vi "qDRC.vi"(0 "System no.":i32=1 min=1 max=4 step=1, 2 "Rec. table to query":i32[](array[numeric]), 3 "With Rec. table IDs?":bool, 5 "error in":errorcluster) -> (14 "Rec. option":i32[](array[numeric]), 15 "Source ID":string[](array[string]), 16 "Trigger option":i32[](array[numeric]), 19 "error out":errorcluster)   [LabVIEW 2020]
doc: "Returns the data recording configuration (Source ID and Rec. option) for the queried record table. \nGCS 2.0: Trigger option is not valid.\n\nC-413, C-843, C-866. C-867, C-877, C-886, C-887, C-891, E-517,E-518,E-709, E-712, E-725, E-727, E-753, E-754, E-861, E-871, E-873, E-874, F-206, M-8X0, Mercury_GCS: Trigger option is not valid.\n\nC-887, F-206, M-8X0: Only for GCS syntax version = GCS 2.0 or higher (check with CSV?.vi. If CSV?.vi is not supported, syntax version is GCS 1.0)."
panel:
  # "Returns the data recording configuration (Source ID, Rec. option and Trigger opt.) for the queried \nrecord tables. GCS 2.0: Trigger option is not valid."
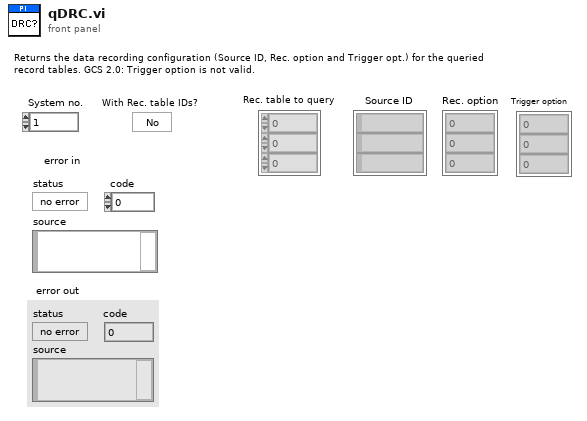
[diagram p1: front panel]
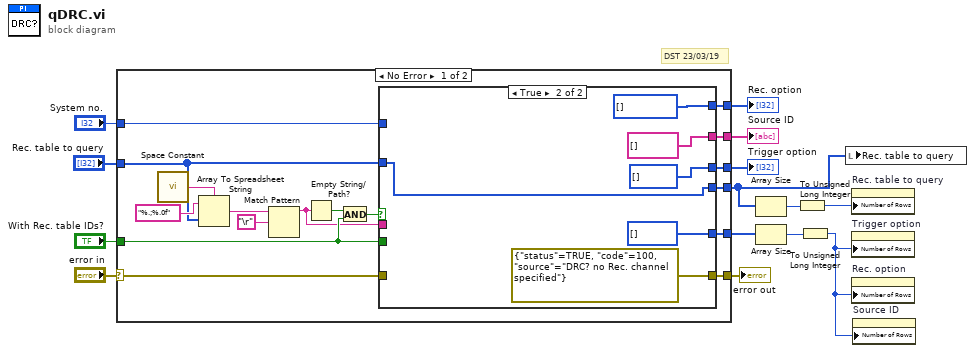
[diagram p0: block diagram]
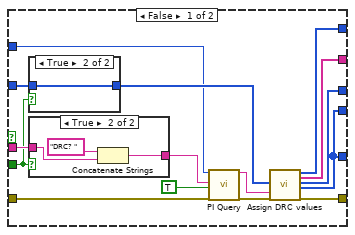
[diagram p2: hidden frame]
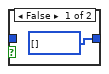
[diagram p3: hidden frame]
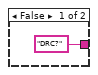
[diagram p4: hidden frame]
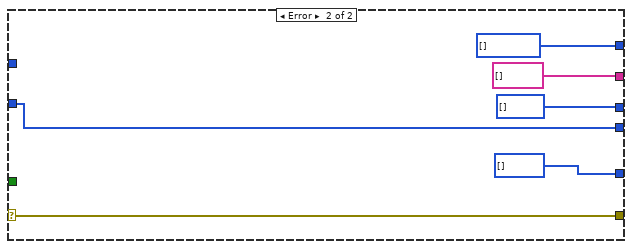
[diagram p5: hidden frame]
diagram:
  # "DST 23/03/19"
  n1 = case shown="No Error" "error in" {
    selector: "error in" -> [w17 w61]
    tunnel: "Rec. table to query" -> [w23 w59]
    tunnel: "System no." -> [w29 _]
    tunnel: [w31 w61] -> w12
    tunnel: [w30 i32[] [] ("Parameter values")] -> w11
    tunnel: [w24 string[] [] ("Source ID")] -> w10
    tunnel: "With Rec. table IDs?" -> [w20 _]
    tunnel: [w21 i32[] [] ("Trigger option")] -> w8
    tunnel: [w16 i32[] [] ("Queried Rec. table out")] -> w5
    tunnel: [w15 w59] -> w3
    frame No Error {
      n2 = call <vilib>:"Space Constant.vi"() -> ("String"=w27:string)
      n3 = Array To Spreadsheet String(delimiter (Tab)=w27, array=w23, 3:"%.;%.0f" ("Format String")) -> (spreadsheet string=w25:string)
      n4 = Match Pattern(string=w25, regular expression="\r") -> (before substring=w19:string)  [unwired: 4 out]
      n5 = Empty String/Path?(string/path=w19) -> (empty?=w18:bool)
      n6 = And(x=w18, y=w20) -> (x .and. y?=w22:bool)
      n7 = case shown="True" w22 {
        tunnel: w17 -> [w43 _]
        tunnel: w19 -> [w44 _]
        tunnel: w29 -> [w34 _]
        tunnel: [w40 errorcluster {"status"=TRUE, "code"=100, "source"="DRC? no Rec. channel specified"} ("error out")] -> w31
        tunnel: [w42 i32[] [] ("Parameter values")] -> w30
        tunnel: [w41 string[] [] ("Source ID")] -> w24
        tunnel: w23 -> [w38 w53]
        tunnel: [w39 i32[] [] ("Trigger option")] -> w21
        tunnel: w20 -> [w33 _]
        tunnel: [w32 i32[] [] ("Queried Rec. table out")] -> w16
        tunnel: [w32 w53] -> w15
        frame False {
          n8 = case shown="True" w33 {
            tunnel: [i32[] [] ("Rec. table to query") w48] -> w37
            tunnel: w38 -> [_ w48]
            frame False {
            }
            frame True {
            }
          }
          n9 = case shown="True" w33 {
            tunnel: ["DRC?" w51] -> w45
            tunnel: w44 -> [_ w50]
            frame False {
            }
            frame True {
              n10 = Concatenate Strings("DRC? ", w50) -> (w51:string)
            }
          }
          n11 = call "PI Query.vi"("System no."=w34, "String to send"=w45, "Attach termination char.?"=TRUE ("Attach Linefeed?"), "error in"=w43) -> ("String read"=w36:string, "error out"=w35:errorcluster)  [unwired: 3 in, 11 out]
          n12 = call "Assign DRC values.vi"("Queried Rec. table"=w37, "Input String"=w36, "error in"=w35) -> ("Rec. option"=w42:i32[], "Source ID"=w41:string[], "Trigger option"=w39:i32[], "Queried Rec. table out"=w32:i32[], "error out"=w40:errorcluster)  [unwired: 1 in, 11 out]
        }
        frame True {
        }
      }
    }
    frame Error {
    }
  }
  "Source ID" <- w10
  "error out" <- w12
  "Rec. option" <- w11
  "Trigger option" <- w8
  n13 = Array Size(array=w3) -> (size(s)=w2:i32)
  n14 = Array Size(array=w5) -> (size(s)=w6:i32)
  n15 = To Unsigned Long Integer(number=w2) -> (unsigned 32bit integer=w1:u32)
  n16 = To Unsigned Long Integer(number=w6) -> (unsigned 32bit integer=w4:u32)
  n17 = local write "Rec. table to query"(w3) -> ()
  n18 = property on="Rec. table to query" class="Arr (strict)"("Number of Rows"=w1) -> ()  [unwired: 2 in, 2 out]
  n19 = property on="Trigger option" class="Arr (strict)"("Number of Rows"=w4) -> ()  [unwired: 2 in, 2 out]
  n20 = property on="Rec. option" class="Arr (strict)"("Number of Rows"=w4) -> ()  [unwired: 2 in, 2 out]
  n21 = property on="Source ID" class="Arr (strict)"("Number of Rows"=w4) -> ()  [unwired: 2 in, 2 out]
